vi "setDPOS.vi"(8 "error in (no error)":errorcluster, 9 "DPOS In Current Units":dbl, 10 "Axis Letter":string, 11 "Controller in":refnum<class "Controller.lvclass">) -> (0 "error out":errorcluster, 3 "Controller out":refnum<class "Controller.lvclass">)   [LabVIEW 2019, in "Controller.lvclass"]
uses:
  Controller.lvclass
  Axis/Axis.lvclass
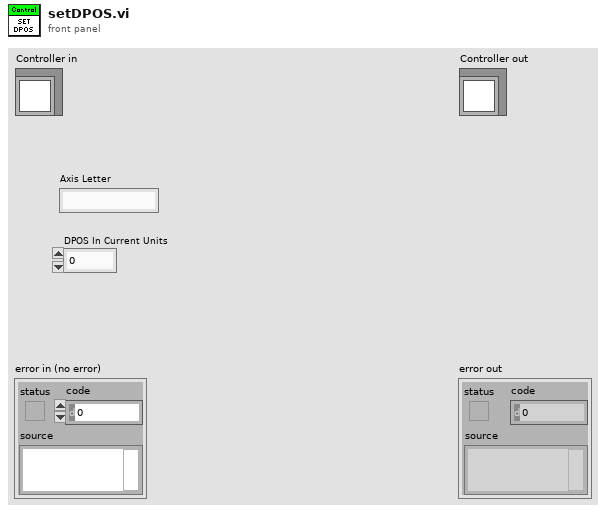
[diagram p1: front panel]
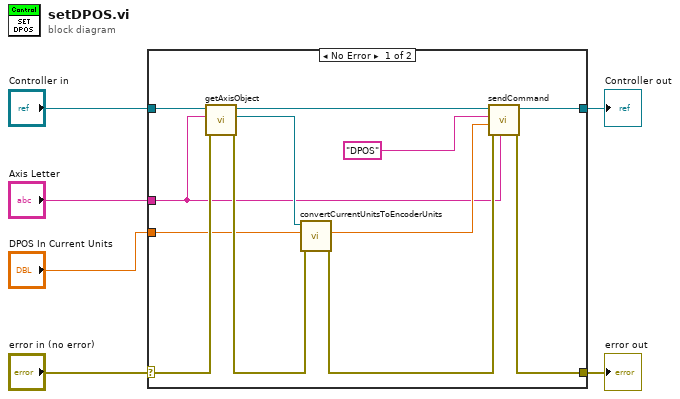
[diagram p0: block diagram]
diagram:
  n1 = case shown="No Error" "error in (no error)" {
    selector: "error in (no error)" -> [w17 w20]
    tunnel: [w13 w20] -> w5
    tunnel: [w11 w19] -> w3
    tunnel: "Controller in" -> [w18 w19]
    tunnel: "Axis Letter" -> [w7 _]
    tunnel: "DPOS In Current Units" -> [w8 _]
    frame No Error {
      n2 = call-dynamic "getAxisObject.vi"("error in (no error)"=w17, "Axis Letter"=w7, "Controller in"=w18) -> ("error out"=w12:errorcluster, "Axis Object"=w16:refnum<class "Axis.lvclass">, "Controller out"=w15:refnum<class "Controller.lvclass">)  [unwired: 6 in]
      n3 = call-dynamic "convertCurrentUnitsToEncoderUnits.vi"("error in (no error)"=w12, "Value In Current Units"=w8, "Axis in"=w16) -> ("error out"=w14:errorcluster, "Value In Encoder Units"=w9:dbl)  [unwired: 6 in, 1 out]
      n4 = call-dynamic "sendCommand.vi"("Axis Letter"=w7, "error in (no error)"=w14, "Value"=w9, "Command"="DPOS", "Controller in"=w15) -> ("error out"=w13:errorcluster, "Controller out"=w11:refnum<class "Controller.lvclass">)  [unwired: 5 in]
    }
    frame Error {
    }
  }
  "error out" <- w5
  "Controller out" <- w3
